vi "Send Message.vi"(8 "error in (no error)":errorcluster, 10 "Message":T1={"Command"="", "Data"=variant(string ""), "ID"="", "error"={"status"=FALSE, "code"=0, "source"=""}}, 11 "RemoteControl in":refnum<class "RemoteControl.lvclass">) -> (0 "error out":errorcluster, 3 "RemoteControl out":refnum<class "RemoteControl.lvclass">)   [LabVIEW 2019, in "RemoteControl.lvlib" / "RemoteControl.lvclass"]
uses:
  RemoteControl.lvclass
  Typedefs/Message--Cluster.ctl
  RemoteControl.lvclass/RemoteControl.ctl
  Private/RemoteControl.GlobalVariable.vi
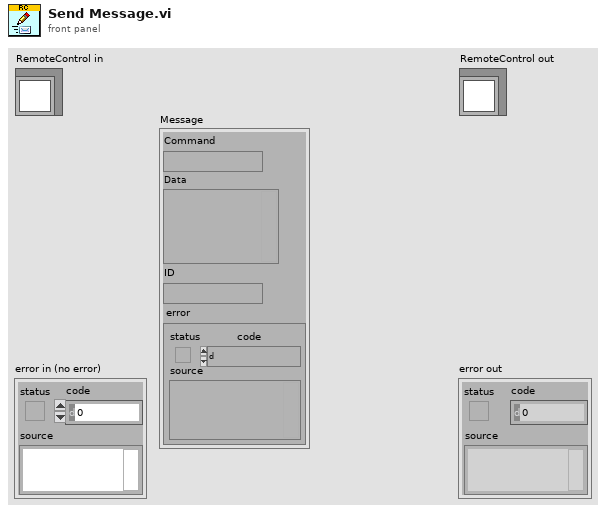
[diagram p1: front panel]
types:
  T1 = typedef "RemoteControl.lvlib/RemoteControl.lvclass/Message--Cluster.ctl" = cluster{"Command":string, "Data":variant, "ID":string, "error":errorcluster}
  T2 = typedef "RemoteControl.lvlib/RemoteControl.lvclass/RC Process Type--Enum.ctl" = enum16{"Listener", "Server", "Client"}
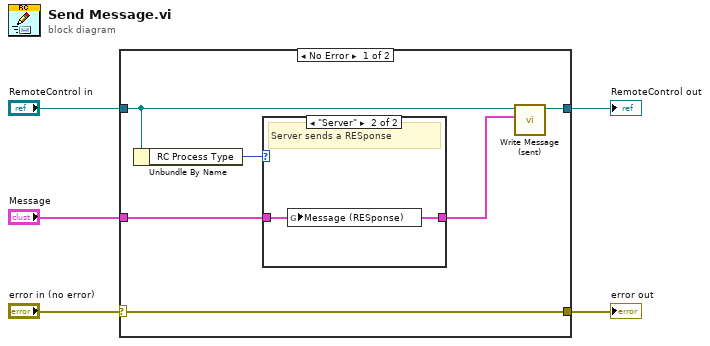
[diagram p0: block diagram]
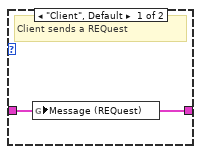
[diagram p2: hidden frame]
diagram:
  n1 = case shown="No Error" "error in (no error)" {
    selector: "error in (no error)" -> [w7 w15]
    tunnel: [w7 w15] -> w5
    tunnel: [w11 w14] -> w3
    tunnel: "RemoteControl in" -> [w9 w14]
    tunnel: "Message" -> [w10 _]
    frame No Error {
      n2 = Unbundle By Name(w9) -> ("RC Process Type"=w8:T2)
      n3 = case shown="\"Server\"" w8 {
        tunnel: w10 -> [w12 w13]
        tunnel: [w12 w13] -> w6
        frame "Client", Default {
          # "Client sends a REQuest"
          n4 = global write "RemoteControl.GlobalVariable.vi" "Message (REQuest)"(w12) -> ()
        }
        frame "Server" {
          # "Server sends a RESponse"
          n5 = global write "RemoteControl.GlobalVariable.vi" "Message (RESponse)"(w13) -> ()
        }
      }
      n6 = call "Write Message (sent).vi"("Message"=w6, "RemoteControl in"=w9) -> ("RemoteControl out"=w11:refnum<class "RemoteControl.lvclass">)  [unwired: 9 in]
    }
    frame Error {
    }
  }
  "error out" <- w5
  "RemoteControl out" <- w3
